vi "Create_Trajectory_Using_PathfinderDifferential_NAT.vi"() -> ()   [LabVIEW 2019]
uses:
  <vilib>/Rock Robotics/WPI/ThirdParty/JAS_Junk/JaciPathFinderLib/VIs/Waypoint.ctl
  <vilib>/Rock Robotics/WPI/ThirdParty/JAS_Junk/TrajLib/TRAJ_STATE.ctl
  <vilib>/Rock Robotics/WPI/ThirdParty/JAS_Junk/TrajLib/POSE2D.ctl
  <vilib>/Rock Robotics/WPI/ThirdParty/JAS_Junk/TrajLib/TRANSLATION2D.ctl
  <vilib>/Rock Robotics/WPI/ThirdParty/JAS_Junk/TrajLib/ROTATION2D.ctl
  <vilib>/Utility/miscctls.llb/LVCursorListTypeDef.ctl
  <vilib>/Rock Robotics/WPI/ThirdParty/JAS_Junk/TrajLib/UTIL_PATHFINDER_CONFIG.ctl
  <vilib>/Rock Robotics/WPI/ThirdParty/JAS_Junk/TrajLib/DISPLAY_WAYPOINT.ctl
  <vilib>/Utility/inputDevices.llb/mouseAcquire.vi
  <vilib>/Rock Robotics/WPI/ThirdParty/JAS_Junk/JaciPathFinderLib/Pathfinder.lvlib
  <vilib>/Rock Robotics/WPI/ThirdParty/JAS_Junk/TrajLib/Trajectory_Library.lvlib
panel:
  out "CursIdx":i32
  out "Cursor Update Mode":i32=1
  out "Angle":dbl
  out "Scrolling":i32
  out "Index":i32
  in  "End Program":bool
  in  "Tab Control":T1(tab)
  in  "max_velocity":dbl=58.0
  in  "max_acceleration":dbl=65.0
  in  "max_jerk":dbl=70.0
  in  "wheelbase_width":dbl=20.866
  in  "Real max\n speed":dbl=65.0
  out "Position":cluster{dbl[], dbl[]}[](graph)
  in  "Waypoints":T2[](array[typedef])=[{"x"=15.0, "y"=105.0, "angle"=-45.0}, {"x"=105.0, "y"=65.0, "angle"=0.0}, {"x"=210.0, "y"=106.0, "angle"=45.0}]
  in  "Path Results\ndT":dbl=0.02 format="%7.3f"
  in  "sample_count":i32=100000
  out "Path calculation error":errorcluster
  out "Complete,\nReady to \nSave file":bool
  out "Path \nSpeed > \nMax":bool
  out "max speed":dbl
  in  "Remove Cursor":bool
  in  "Add Cursor":bool
  in  "Calculate\nPath":bool
  out "Path Data":cluster{dbl[], dbl[]}[](graph)
  out "Traj States\nSize":i32
  out "Trajectory States":T3[](array[typedef]) {"POSE"."ROTATION"."SIN" format="%13.4f"; "POSE"."ROTATION"."COS" format="%13.4f"; "POSE"."ROTATION"."VALUE" format="%13.4f"; "POSE"."TRANSLATION"."Y" format="%14.3f"; "POSE"."TRANSLATION"."X" format="%14.3f"}
  out "File Saved\nWithout\nError":bool
  in  "Trajectory Type":enum32{"Radio Selection 1", "Radio Selection 2"}(radio)
  out "File Creation\nError":errorcluster
  in  "Trajectory File Comment":string
  in  "Trajectory File Name":path
  in  "CreateCmdList":bool
  # "Create trajectory using \"Jaci's Pathfinder\"  (Display for differential drive robot)"
  # "Instructions:\n----------------  \nThis utility will create a trajectory,, show the data on the various tabs, and optionally write a \"robot relative\" trajectory to a \nfile. To use this utility:\n\n1) Read all of these instructions!\n2) Define the Robot Data. on the \"Robot Data\" tab.\n3) Define the \"Path Definition\" on the \"Define / Create Trajectory\" tab.  These are the beginning and ending positions/headings, and \n     internal positions/headings.\n4) Define the time increment.  0.020 is chosen since that matches the normal robot loop time.\n5) Define \"sample count\".  This is an internal PathFinder variable.  Leaving the value as default should work correctly.  Making \n    the value a little smaller will speed the program up a little.\n6) Press the \"Calculate Path\".  If a good path was calculated it will be displayed on the \"Field Position tab, and the \"Complete, \n    Ready to Save\" indicator will light.  The path can be recalculated many times before performing any other action.\n\nAfter a Path has been calculated, the \"trajectory can be written to a file.  The absolute path is converted to a robot relative \ntrajectory.  To do this:\n1) Enter a comment to be included in the file.  Anything can be entered.\n2) Select the file name.\n3) Select the type of trajectory to save, absolute or relative.\n4) Press \"Create Trajectory File\"  If an error occurs it will be displayed in the File Creation Error indicator.\n\nNotes:\n---------\n- All the robot parameters, path, and field dimensions are in INCHES, and DEGREES.  The resulting trajectory is converted to \n   METERS, and RADIANS to match the rest of this library!\n- The pathfinder path generation logic doesn't account distribution of speed to the left and right wheels.  As a result the \n   maximum speed can be exceeded.If this happens, but Path Speed > Max light will light and Ready to Execute will not \n   light.  Lower the maximum speed in the Robot Data tab and recalulate the path.  (CURRENTLY THIS LOGIC IS NOT COMPLETE.)\n- 2019 playing field size - width: 26 ft 11.25 In = 323.25 in , length: 52 ft 5.25 in = 629.25 in  (I didn't verify this for the 2020 version.)"
  # "ROBOT DATA"
  # "INCHES/SEC"
  # "INCHES/SEC"
  # "INCHES/SEC^2"
  # "INCHES/SEC^3"
  # "Simulated robot wheelbase is: 20.866"
  # "INCHES"
  # "Simulated robot max speed is: 68.266"
  # "SEC"
  # "PATH DEFINITION"
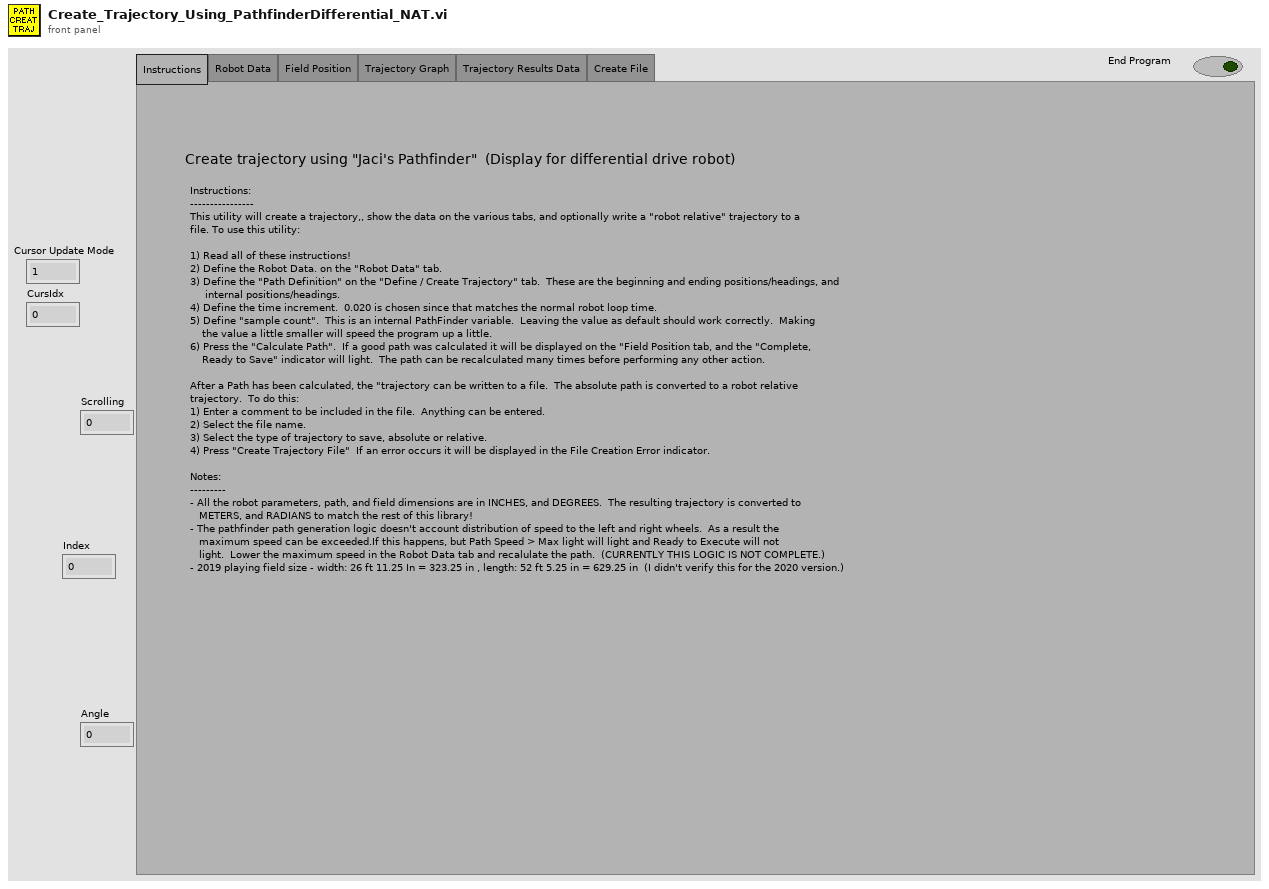
[diagram p1: front panel]
types:
  T1 = enum32{"Instructions", "Robot Data", "Field Position", "Trajectory Graph", "Trajectory Results Data", "Create File"}
  T2 = typedef "Pathfinder.lvlib/Waypoint.ctl" = cluster{"x":dbl, "y":dbl, "angle":dbl}
  T3 = typedef "Trajectory_Library.lvlib/TRAJ_STATE.ctl" = cluster{"TimeSeconds":dbl, "Velocity":dbl, "Acceleration":dbl, "POSE":T4, "Curvature":dbl}
  T4 = typedef "Trajectory_Library.lvlib/POSE2D.ctl" = cluster{"TRANSLATION":T5, "ROTATION":T6}
  T5 = typedef "Trajectory_Library.lvlib/TRANSLATION2D.ctl" = cluster{"X":dbl, "Y":dbl}
  T6 = typedef "Trajectory_Library.lvlib/ROTATION2D.ctl" = cluster{"VALUE":dbl, "COS":dbl, "SIN":dbl}
  T7 = typedef "LVCursorListTypeDef.ctl" = cluster{"Name":string, "Color":u32, "Style":u8, "Point Style":u8, "Name Visible":bool, "Allow Drag":bool, "Cursor Mode":u32, "Plot":i32, "Index":i32, "Position":cluster{"X":dbl, "Y":dbl}, "X Scale":u32, "Y Scale":u32, "Watch Plots":i32[], "Watch All Plots":bool, "Plot Area":i32, "Label Offset":cluster{"X":dbl, "Y":dbl}}[]
  T8 = typedef "Trajectory_Library.lvlib/DISPLAY_WAYPOINT.ctl" = cluster{"X":dbl, "Y":dbl, "ANGLE":dbl}
  T9 = cluster{"Name":string, "Color":u32, "Style":u8, "Point Style":u8, "Name Visible":bool, "Allow Drag":bool, "Cursor Mode":u32, "Plot":i32, "Index":i32, "Position":cluster{"X":dbl, "Y":dbl}, "X Scale":u32, "Y Scale":u32, "Watch Plots":i32[], "Watch All Plots":bool, "Plot Area":i32, "Label Offset":cluster{"X":dbl, "Y":dbl}}
  T10 = typedef "Trajectory_Library.lvlib/UTIL_PATHFINDER_CONFIG.ctl" = cluster{"PathfinderType - 0 tank 1 serve":i32, "PathMaxVelocity - inches per sec":dbl, "MaxAcceleration - inches per sec2":dbl, "MaxJerk--Inches per sec2":dbl, "TimeDelta-Seconds":dbl, "SampleCount":i32, "WheelbaseWidth-inches":dbl, "WheelbaseDepth-inches":dbl, "SwerveType":i32, "ActualMaxVelocity-inches per sec":dbl}
  T11 = cluster{"Horizontal":i32, "Vertical":i32, "Scrolling":i32}
  T12 = typedef "Trajectory_Library.lvlib/TRAJECTORY.ctl" = cluster{"TotalTImeSecs":dbl, "States":T3[]}
  T13 = typedef "Pathfinder.lvlib/Segment.ctl" = cluster{"dt":dbl, "x":dbl, "y":dbl, "position":dbl, "velocity":dbl, "acceleration":dbl, "jerk":dbl, "heading":dbl}
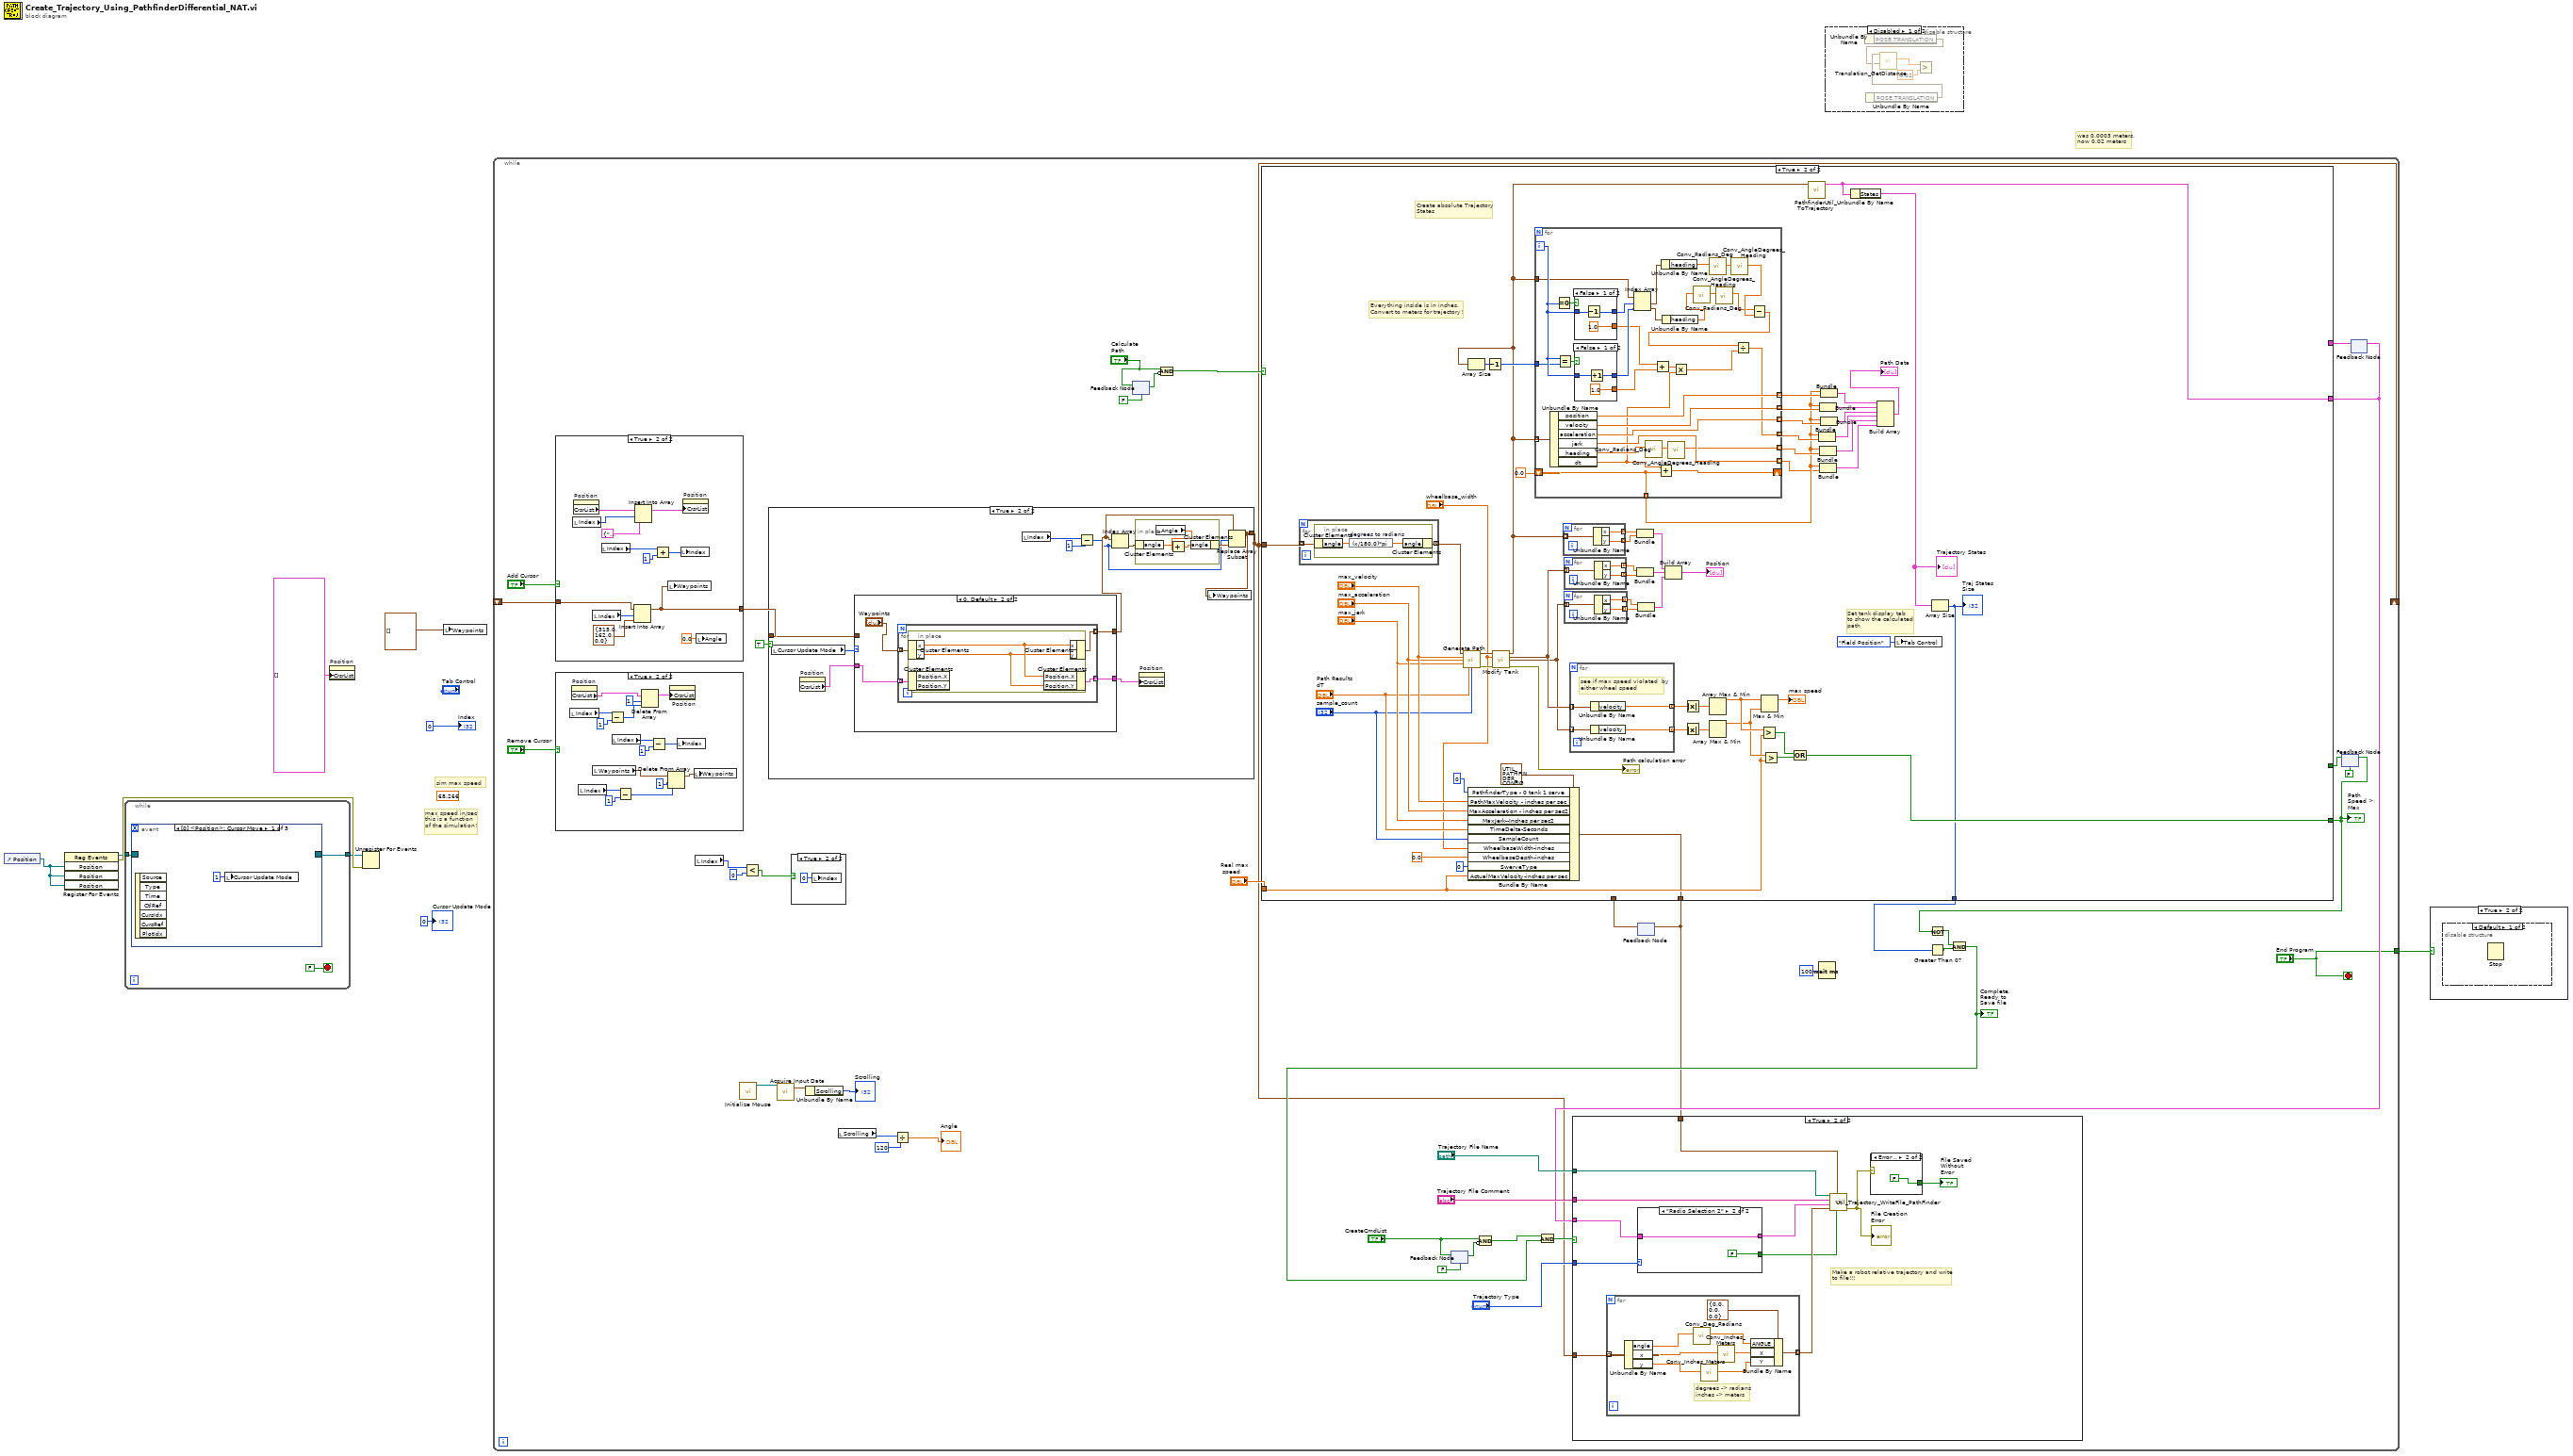
[diagram p0: block diagram]
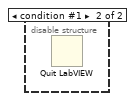
[diagram p3: hidden frame]
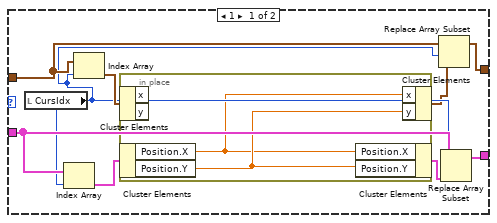
[diagram p5: hidden frame]
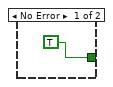
[diagram p9: hidden frame]
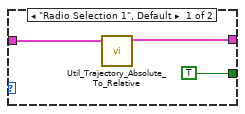
[diagram p10: hidden frame]
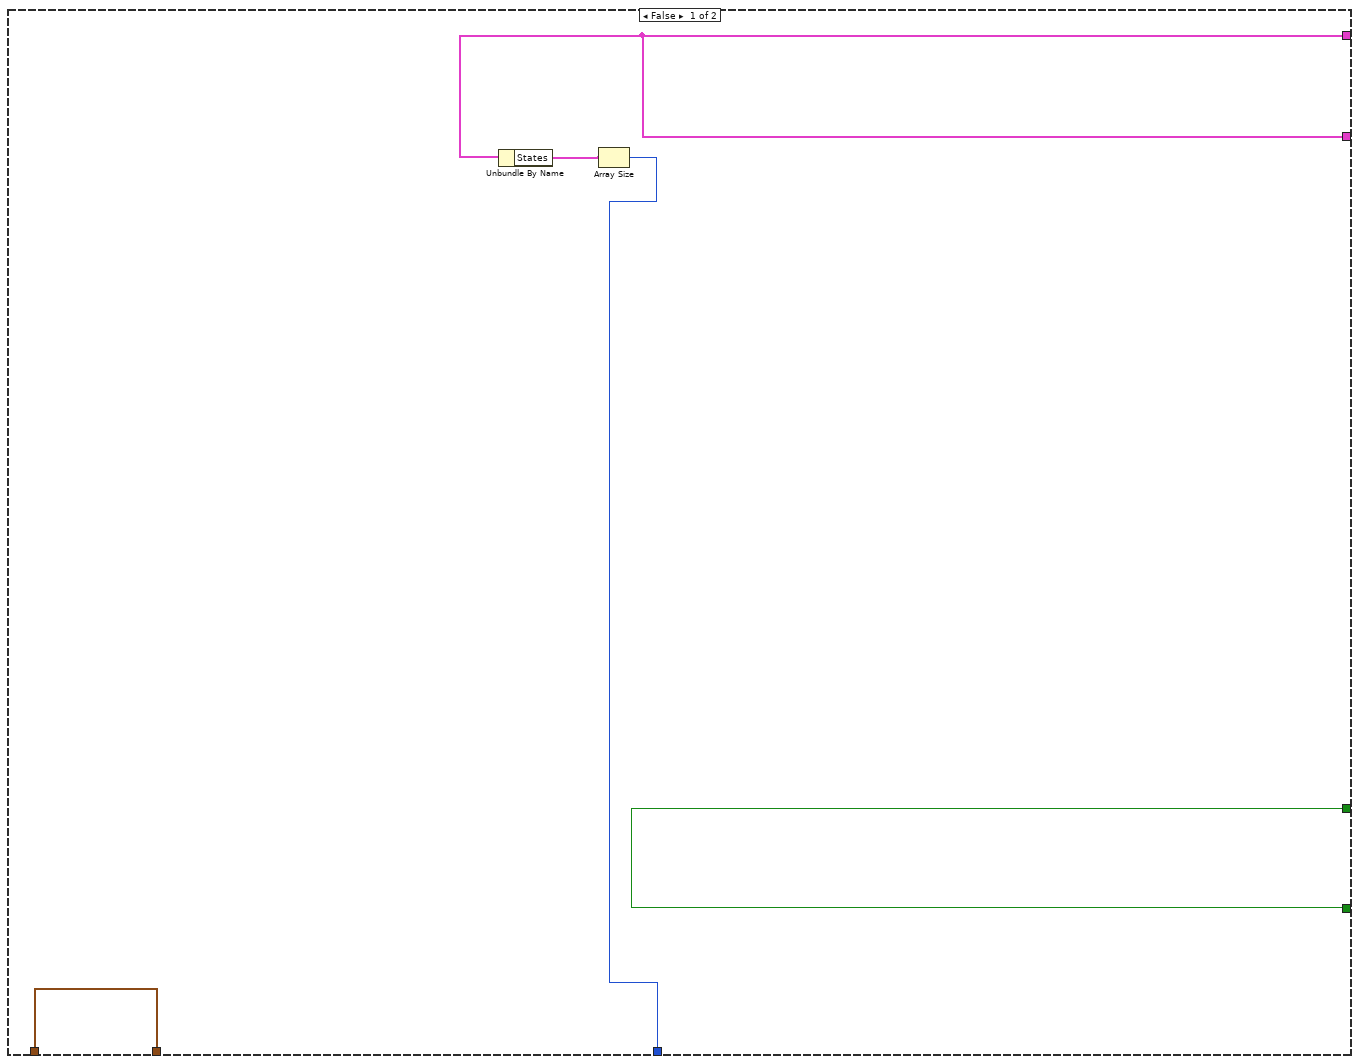
[diagram p12: hidden frame]
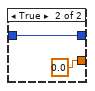
[diagram p13: hidden frame]
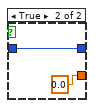
[diagram p14: hidden frame]
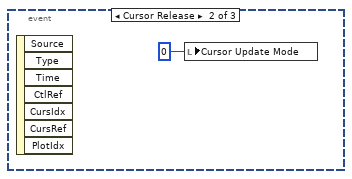
[diagram p15: hidden frame]
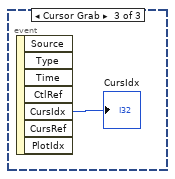
[diagram p16: hidden frame]
diagram:
  (unwired) 68.266 ("x")
  # "was 0.0003 meters.\nnow 0.02 meters"
  # "sim max speed"
  # "max speed in/sec\nthis is a function\nof the simulation!"
  n1 = control-ref of="Position"() -> (w4:refnum<vi>)
  n2 = register-events(w4, w4, w4) -> (reference out=w5:refnum<event-registration>, error out=w7:errorcluster)  [unwired: 2 in]
  n3 = while {
    tunnel: w5 -> [w12]
    tunnel: [w11] -> w6
    stop <- FALSE stop-if-true
    n4 = event shown="[0] <Position>: Cursor Move" {
      selector: w12 -> [_ _ _]
      dyn-events: [_ _ _] -> w11
      timeout: _ -> [_ _ _]
      event Cursor Move {
        n5 = event-data() -> ()  [unwired: 1 in, 7 out]
        n6 = local write "Cursor Update Mode"(1 ("Cursor Update Mode")) -> ()
      }
      event Cursor Release {
        n7 = event-data() -> ()  [unwired: 1 in, 7 out]
        n8 = local write "Cursor Update Mode"(0 ("Wapoint Update Mode")) -> ()
      }
      event Cursor Grab {
        n9 = event-data() -> ("CursIdx"=→"CursIdx":i32)  [unwired: 1 in, 6 out]
      }
    }
  }
  n10 = property on="Position" class="XYGraph (strict)"("CrsrList"=T7 [] ("Cursor List")) -> ()  [unwired: 2 in, 2 out]
  n11 = Unregister For Events(event registration refnum=w6, error in=w7) -> ()  [unwired: 1 out]
  n12 = local write "Waypoints"(T2[] [] ("Waypoints")) -> ()
  n13 = while {
    tunnel: ["End Program"] -> w9
    shift-right: [w17] -> _
    shift-left: _ -> [w22]
    stop <- "End Program" stop-if-true
    n14 = case shown="True" "Add Cursor" {
      tunnel: w22 -> [w136 w140]
      tunnel: [w136 w138] -> w18
      frame False {
      }
      frame True {
        n15 = local read "Index"() -> (w146:i32)
        n16 = property on="Position" class="XYGraph (strict)"() -> ("CrsrList"=w148:T7)  [unwired: 2 in, 2 out]
        n17 = local read "Index"() -> (w142:i32)
        n18 = local read "Index"() -> (w144:i32)
        n19 = Insert Into Array(array=w140, index=w142, new element=T2 {"x"=315.0, "y"=162.0, "angle"=0.0} ("new element/subarray")) -> (w138:T2[])
        n20 = Insert Into Array(array=w148, index=w146, new element=T9 {"Name"="Cursor", "Color"=5635906, "Style"=4, "Point Style"=2, "Name Visible"=FALSE, "Allow Drag"=TRUE, "Cursor Mode"=0, "Plot"=0, "Index"=0, "Position"={"X"=315.0, "Y"=162.0}, "X Scale"=0, "Y Scale"=0, "Watch Plots"=[], "Watch All Plots"=FALSE, "Plot Area"=0, "Label Offset"={"X"=0.0, "Y"=0.0}} ("new element/subarray")) -> (w147:T7)
        n21 = Add(x=w144, y=1) -> (x+y=w143:i32)
        n22 = local write "Waypoints"(w138) -> ()
        n23 = local write "Index"(w143) -> ()
        n24 = property on="Position" class="XYGraph (strict)"("CrsrList"=w147) -> ()  [unwired: 2 in, 2 out]
        n25 = local write "Angle"(0.0 ("Angle")) -> ()
      }
    }
    n26 = case shown="True" "Remove Cursor" {
      frame False {
      }
      frame True {
        n27 = local read "Index"() -> (w104:i32)
        n28 = property on="Position" class="XYGraph (strict)"() -> ("CrsrList"=w99:T7)  [unwired: 2 in, 2 out]
        n29 = local read "Index"() -> (w103:i32)
        n30 = local read "Waypoints"() -> (w95:T2[])
        n31 = Subtract(x=w104, y=1) -> (x-y=w101:i32)
        n32 = local read "Index"() -> (w107:i32)
        n33 = Subtract(x=w103, y=1) -> (x-y=w97:i32)
        n34 = Delete From Array(array=w99, length=1, index=w101) -> (array with subset deleted=w98:T7)  [unwired: 1 out]
        n35 = Subtract(x=w107, y=1) -> (x-y=w108:i32)
        n36 = Delete From Array(array=w95, length=1, index=w97) -> (array with subset deleted=w94:T2[])  [unwired: 1 out]
        n37 = property on="Position" class="XYGraph (strict)"("CrsrList"=w98) -> ()  [unwired: 2 in, 2 out]
        n38 = local write "Index"(w108) -> ()
        n39 = local write "Waypoints"(w94) -> ()
      }
    }
    n40 = local read "Index"() -> (w21:i32)
    n41 = call <vilib>:"Initialize Mouse.vi"() -> ("device ID"=w28:refnum<k1>)  [unwired: 10 in, 1 out]
    n42 = Less?(x=w21, y=0) -> (x < y?=w19:bool)
    n43 = case shown="True" TRUE {
      tunnel: w18 -> [w57 w67]
      tunnel: [w57 w58] -> w17
      frame False {
      }
      frame True {
        n44 = local read "Cursor Update Mode"() -> (w68:i32)
        n45 = property on="Position" class="XYGraph (strict)"() -> ("CrsrList"=w66:T7)  [unwired: 2 in, 2 out]
        n46 = case shown="0, Default" w68 {
          tunnel: w66 -> [w75 w86]
          tunnel: w67 -> [w78 _]
          tunnel: [w77 w85] -> w61
          tunnel: [w73 w84] -> w65
          frame 1 {
            n47 = local read "CursIdx"() -> (w74:i32)
            n48 = Index Array(array=w75, index=w74) -> (element=w80:T9)
            n49 = Index Array(array=w78, index=w74) -> (element=w79:T2)
            n50 = in-place {
              n51 = in-place-cluster #1(w79) -> ()  [unwired: 2 out]
              n52 = in-place-cluster #2(w80) -> ("Position.X"=w81:dbl, "Position.Y"=w82:dbl)
              n53 = in-place-cluster #2("Position.X"=w81, "Position.Y"=w82) -> (w76:T9)
              n54 = in-place-cluster #1("x"=w81, "y"=w82) -> (w72:T2)
            }
            n55 = Replace Array Subset(array=w78, new element=w72, index=w74) -> (w77:T2[])
            n56 = Replace Array Subset(array=w75, new element=w76, index=w74) -> (w73:T7)
          }
          frame 0, Default {
            n57 = for {
              tunnel: w86 -> [w90] mode=indexing
              tunnel: "Waypoints" -> [w89] mode=indexing
              tunnel: [w88] -> w85 mode=indexing
              tunnel: [w87] -> w84 mode=indexing
              n58 = in-place {
                n59 = in-place-cluster #3(w89) -> ("x"=w92:dbl, "y"=w91:dbl)
                n60 = in-place-cluster #4(w90) -> ()  [unwired: 2 out]
                n61 = in-place-cluster #4("Position.X"=w92, "Position.Y"=w91) -> (w87:T9)
                n62 = in-place-cluster #3("x"=w92, "y"=w91) -> (w88:T2)
              }
            }
          }
        }
        n63 = local read "Index"() -> (w60:i32)
        n64 = Subtract(x=w60, y=1) -> (x-y=w59:i32)
        n65 = Index Array(array=w61, index=w59) -> (element=w62:T2)
        n66 = in-place {
          n67 = in-place-cluster #5(w62) -> ("angle"=w71:dbl)
          n68 = local read "Angle"() -> (w70:dbl)
          n69 = Add(x=w70, y=w71) -> (x+y=w69:dbl)
          n70 = in-place-cluster #5("angle"=w69) -> (w64:T2)
        }
        n71 = property on="Position" class="XYGraph (strict)"("CrsrList"=w65) -> ()  [unwired: 2 in, 2 out]
        n72 = Replace Array Subset(array=w61, new element=w64, index=w59) -> (w58:T2[])
        n73 = local write "Waypoints"(w58) -> ()
      }
    }
    n74 = call-poly <vilib>:"Acquire Input Data.vi"("device ID"=w28) -> ("axis info"=w27:T11)  [unwired: 15 in, 3 out]
    n75 = case shown="True" w19 {
      frame False {
      }
      frame True {
        n76 = local write "Index"(0 ("Index")) -> ()
      }
    }
    n77 = Unbundle By Name(w27) -> ("Scrolling"=→"Scrolling":i32)
    n78 = local read "Scrolling"() -> (w23:i32)
    n79 = Divide(x=w23, y=120) -> (x/y=→"Angle":dbl)
    n80 = feedback #6(FALSE ("CreateCmdList")) -> (w39:bool)
    n81 = feedback-in #6("Calculate\nPath") -> ()
    n82 = Compound Arithmetic op=AND("Calculate\nPath", invert w39) -> (w36:bool)
    n83 = feedback-in #7("CreateCmdList") -> ()
    n84 = feedback #7(FALSE ("CreateCmdList")) -> (w42:bool)
    n85 = Compound Arithmetic op=AND("CreateCmdList", invert w42) -> (w41:bool)
    n86 = feedback #8() -> (w31:T10)  [unwired: 1 in]
    n87 = Wait (ms)(milliseconds to wait=u32 100) -> ()  [unwired: 1 out]
    n88 = feedback #9(FALSE) -> (w54:bool)
    n89 = feedback #10() -> (w50:T12)  [unwired: 1 in]
    n90 = case shown="True" w36 {
      tunnel: "Real max\n speed" -> [_ w158]
      tunnel: [w153 w199] -> w51
      tunnel: w54 -> [w153 _]
      tunnel: w17 -> [_ w198]
      tunnel: [w150 w175] -> w45
      tunnel: w50 -> [w150 _]
      tunnel: [w152 w190] -> w44
      tunnel: [w149 w154] -> w32
      tunnel: w31 -> [w149 _]
      frame False {
        n91 = Unbundle By Name(w150) -> ("States"=w151:T3[])
        n92 = Array Size(array=w151) -> (size(s)=w152:i32)
      }
      frame True {
        # "Everything inside is in inches.\nConvert to meters for trajectory!"
        # "Create absolute Trajectory\nStates"
        # "Set tank display tab\nto show the calculated\npath"
        n93 = for {
          tunnel: w198 -> [w220] mode=indexing
          tunnel: [w219] -> w212 mode=indexing
          n94 = in-place {
            n95 = in-place-cluster #11(w220) -> ("angle"=w222:dbl)
            n96 = expression code="(x/180.0)*pi" "degrees to radians"(w222) -> (w221:dbl)
            n97 = in-place-cluster #11("angle"=w221) -> (w219:T2)
          }
        }
        n98 = call <vilib>:"Generate Path.vi"("path"=w212, "max_velocity"="max_velocity", "max_acceleration"="max_acceleration", "max_jerk"="max_jerk", "dt (.001)"="Path Results\ndT", "sample_count (100000)"="sample_count") -> ("Segments"=w213:T13[], "error out"=w202:errorcluster)  [unwired: 8 in]
        n99 = Bundle By Name(cluster=T10 {"PathfinderType - 0 tank 1 serve"=0, "PathMaxVelocity - inches per sec"=0.0, "MaxAcceleration - inches per sec2"=0.0, "MaxJerk--Inches per sec2"=0.0, "TimeDelta-Seconds"=0.0, "SampleCount"=0, "WheelbaseWidth-inches"=0.0, "WheelbaseDepth-inches"=0.0, "SwerveType"=0, "ActualMaxVelocity-inches per sec"=0.0} ("UTIL_PATHFINDER_CONFIG"), "PathfinderType - 0 tank 1 serve"=0, "PathMaxVelocity - inches per sec"="max_velocity", "MaxAcceleration - inches per sec2"="max_acceleration", "MaxJerk--Inches per sec2"="max_jerk", "TimeDelta-Seconds"="Path Results\ndT", "SampleCount"="sample_count", "WheelbaseWidth-inches"="wheelbase_width", "WheelbaseDepth-inches"=0.0, "SwerveType"=0, "ActualMaxVelocity-inches per sec"=w158) -> (w154:T10)
        n100 = call <vilib>:"Modify Tank.vi"("Original"=w213, "wheelbase_width"="wheelbase_width", "error in"=w202) -> ("original"=w166:T13[], "left"=w197:T13[], "right"=w196:T13[], "error out"=→"Path calculation error":errorcluster)  [unwired: 9 in]
        n101 = Array Size(array=w166) -> (size(s)=w168:i32)
        n102 = Decrement(x=w168) -> (x-1=w167:i32)
        n103 = for {
          tunnel: w166 -> [w263] mode=indexing
          shift-right: [w261] -> _
          shift-left: 0.0 -> [w262]
          tunnel: [w262] -> w171 mode=indexing
          tunnel: [w254] -> w172 mode=indexing
          tunnel: [w260] -> w170 mode=indexing
          tunnel: [w259] -> w180 mode=indexing
          tunnel: [w258] -> w179 mode=indexing
          tunnel: [w257] -> w174 mode=indexing
          tunnel: [w240] -> w173 mode=indexing
          tunnel: w166 -> [w246]
          tunnel: w167 -> [w239]
          i -> [w251]
          n104 = Unbundle By Name(w263) -> ("position"=w257:dbl, "velocity"=w258:dbl, "acceleration"=w259:dbl, "jerk"=w260:dbl, "heading"=w256:dbl, "dt"=w242:dbl)
          n105 = Equal To 0?(x=w251) -> (x = 0?=w253:bool)
          n106 = Equal?(x=w251, y=w239) -> (x = y?=w252:bool)
          n107 = case shown="False" w253 {
            tunnel: w251 -> [w271 w272]
            tunnel: [1.0 0.0] -> w243
            tunnel: [w269 w272] -> w248
            frame False {
              n108 = Decrement(x=w271) -> (x-1=w269:i32)
            }
            frame True {
            }
          }
          n109 = case shown="False" w252 {
            tunnel: [1.0 0.0] -> w244
            tunnel: w251 -> [w265 w267]
            tunnel: [w264 w267] -> w247
            frame False {
              n110 = Increment(x=w265) -> (x+1=w264:i32)
            }
            frame True {
            }
          }
          n111 = Index Array(array=w246, index #1=w248, index #2=w247) -> (element #1=w250:T13, element #2=w249:T13)
          n112 = call <vilib>:"Conv_Radians_Deg.vi"("Radians"=w256) -> ("Degrees"=w255:dbl)  [unwired: 10 in]
          n113 = Add(x=w243, y=w244) -> (x+y=w245:dbl)
          n114 = Add(x=w242, y=w262) -> (x+y=w261:dbl)
          n115 = Unbundle By Name(w250) -> ("heading"=w236:dbl)
          n116 = Unbundle By Name(w249) -> ("heading"=w234:dbl)
          n117 = call <vilib>:"Conv_AngleDegrees_Heading.vi"("Degrees"=w255) -> ("Heading Degrees"=w254:dbl)  [unwired: 10 in]
          n118 = Multiply(x=w245, y=w242) -> (x*y=w241:dbl)
          n119 = call <vilib>:"Conv_Radians_Deg.vi"("Radians"=w234) -> ("Degrees"=w233:dbl)  [unwired: 10 in]
          n120 = call <vilib>:"Conv_Radians_Deg.vi"("Radians"=w236) -> ("Degrees"=w237:dbl)  [unwired: 10 in]
          n121 = call <vilib>:"Conv_AngleDegrees_Heading.vi"("Degrees"=w233) -> ("Heading Degrees"=w232:dbl)  [unwired: 10 in]
          n122 = call <vilib>:"Conv_AngleDegrees_Heading.vi"("Degrees"=w237) -> ("Heading Degrees"=w235:dbl)  [unwired: 10 in]
          n123 = Subtract(x=w232, y=w235) -> (x-y=w238:dbl)
          n124 = Divide(x=w238, y=w241) -> (x/y=w240:dbl)
        }
        n125 = for {
          tunnel: w166 -> [w225] mode=indexing
          tunnel: [w224] -> w209 mode=indexing
          tunnel: [w223] -> w210 mode=indexing
          n126 = Unbundle By Name(w225) -> ("x"=w224:dbl, "y"=w223:dbl)
        }
        n127 = for {
          tunnel: w197 -> [w231] mode=indexing
          tunnel: [w230] -> w203 mode=indexing
          tunnel: [w229] -> w204 mode=indexing
          n128 = Unbundle By Name(w231) -> ("x"=w230:dbl, "y"=w229:dbl)
        }
        n129 = for {
          tunnel: w196 -> [w228] mode=indexing
          tunnel: [w227] -> w205 mode=indexing
          tunnel: [w226] -> w206 mode=indexing
          n130 = Unbundle By Name(w228) -> ("x"=w227:dbl, "y"=w226:dbl)
        }
        n131 = for {
          tunnel: w197 -> [w218] mode=indexing
          tunnel: w196 -> [w217] mode=indexing
          tunnel: [w216] -> w195 mode=indexing
          tunnel: [w215] -> w193 mode=indexing
          # "see if max speed violated  by\neither wheel speed"
          n132 = Unbundle By Name(w218) -> ("velocity"=w216:dbl)
          n133 = Unbundle By Name(w217) -> ("velocity"=w215:dbl)
        }
        n134 = Bundle(w209, w210) -> (w211:cluster{dbl[], dbl[]})  [unwired: 1 in]
        n135 = Bundle(w203, w204) -> (w208:cluster{dbl[], dbl[]})  [unwired: 1 in]
        n136 = Bundle(w205, w206) -> (w207:cluster{dbl[], dbl[]})  [unwired: 1 in]
        n137 = Build Array(w211, w208, w207) -> (→"Position":cluster{dbl[], dbl[]}[])
        n138 = Absolute Value(x=w195) -> (abs(x)=w194:dbl[])
        n139 = Absolute Value(x=w193) -> (abs(x)=w192:dbl[])
        n140 = Array Max & Min(array=w194) -> (max value=w189:dbl)  [unwired: 3 out]
        n141 = Array Max & Min(array=w192) -> (max value=w188:dbl)  [unwired: 3 out]
        n142 = Max & Min(x=w189, y=w188) -> (max(x,y)=→"max speed":dbl)  [unwired: 1 out]
        n143 = Greater?(x=w189, y=w158) -> (0:w200:bool)
        n144 = Greater?(x=w188, y=w158) -> (0:w191:bool)
        n145 = Compound Arithmetic op=OR(w200, w191) -> (w199:bool)
        n146 = call <vilib>:"PathfinderUtil_ToTrajectory.vi"("Pathfinder Path"=w166) -> ("TRAJECTORY"=w175:T12)  [unwired: 10 in]
        n147 = Bundle(w171, w173) -> (w183:cluster{dbl[], dbl[]})  [unwired: 1 in]
        n148 = Bundle(w171, w172) -> (w182:cluster{dbl[], dbl[]})  [unwired: 1 in]
        n149 = Bundle(w171, w179) -> (w185:cluster{dbl[], dbl[]})  [unwired: 1 in]
        n150 = Bundle(w171, w170) -> (w169:cluster{dbl[], dbl[]})  [unwired: 1 in]
        n151 = Bundle(w171, w174) -> (w186:cluster{dbl[], dbl[]})  [unwired: 1 in]
        n152 = Bundle(w171, w180) -> (w184:cluster{dbl[], dbl[]})  [unwired: 1 in]
        n153 = Unbundle By Name(w175) -> ("States"=w177:T3[])
        "Trajectory States" <- w177
        n154 = Build Array(w186, w185, w184, w183, w182, w169) -> (→"Path Data":cluster{dbl[], dbl[]}[])
        n155 = local write "Tab Control"(T1."Field Position" ("Tab Control")) -> ()
        n156 = Array Size(array=w177) -> (size(s)=w190:i32)
        "Traj States\nSize" <- w190
      }
    }
    "Path \nSpeed > \nMax" <- w51
    n157 = feedback-in #8(w32) -> ()
    n158 = Not(x=w51) -> (.not. x?=w52:bool)
    n159 = Greater Than 0?(x=w44) -> (x > 0?=w53:bool)
    n160 = And(x=w52, y=w53) -> (x .and. y?=w46:bool)
    "Complete,\nReady to \nSave file" <- w46
    n161 = And(x=w41, y=w46) -> (x .and. y?=w47:bool)
    n162 = case shown="True" w47 {
      tunnel: "Trajectory File Name" -> [_ w119]
      tunnel: "Trajectory File Comment" -> [_ w118]
      tunnel: w45 -> [_ w114]
      tunnel: w17 -> [_ w117]
      tunnel: "Trajectory Type" -> [_ w113]
      tunnel: w32 -> [_ w109]
      frame False {
      }
      frame True {
        # "Make a robot relative trajectory and write\nto file!!!"
        n163 = for {
          tunnel: w117 -> [w135] mode=indexing
          tunnel: [w134] -> w116 mode=indexing
          # "degrees -> radians\ninches -> meters"
          n164 = Unbundle By Name(w135) -> ("angle"=w128:dbl, "x"=w133:dbl, "y"=w131:dbl)
          n165 = call <vilib>:"Conv_Deg_Radians.vi"("Degress"=w128) -> ("Radians"=w129:dbl)  [unwired: 10 in]
          n166 = call <vilib>:"Conv_Inches_Meters.vi"("INCH"=w131) -> ("Meters"=w130:dbl)  [unwired: 10 in]
          n167 = call <vilib>:"Conv_Inches_Meters.vi"("INCH"=w133) -> ("Meters"=w132:dbl)  [unwired: 10 in]
          n168 = Bundle By Name(cluster=T8 {"X"=0.0, "Y"=0.0, "ANGLE"=0.0} ("UTIL_WAYPOINT"), "ANGLE"=w129, "X"=w132, "Y"=w130) -> (w134:T8)
        }
        n169 = case shown="\"Radio Selection 2\"" w113 {
          tunnel: w114 -> [w124 w126]
          tunnel: [w123 w126] -> w115
          tunnel: [TRUE FALSE] -> w110
          frame "Radio Selection 1", Default {
            n170 = call <vilib>:"Util_Trajectory_Absolute_To_Relative.vi"("absTRAJECTORY"=w124) -> ("outputRelativeTRAJECTORY"=w123:T12)  [unwired: 10 in]
          }
          frame "Radio Selection 2" {
          }
        }
        n171 = call <vilib>:"Util_Trajectory_WriteFile_PathFinder.vi"("Trajectory Is Relative"=w110, "UTIL_PATHFINDER_CONFIG"=w109, "UtilityWayPoints"=w116, "TRAJECTORY"=w115, "Comment"=w118, "Trajectory File Name"=w119) -> ("error out"=w112:errorcluster)  [unwired: 5 in]
        "File Creation\nError" <- w112
        n172 = case shown="Error .." w112 {
          tunnel: [TRUE ("File Saved\nWithout\nError") FALSE ("File Saved\nWithout\nError")] -> w111
          frame No Error {
          }
          frame Error {
          }
        }
        "File Saved\nWithout\nError" <- w111
      }
    }
    n173 = feedback-in #9(w51) -> ()
    n174 = feedback-in #10(w45) -> ()
  }
  n175 = disable-structure shown="Disabled" {
    frame Disabled {
      n176 = Unbundle By Name() -> ("POSE.TRANSLATION"=w277:T5)  [unwired: 1 in]
      n177 = Unbundle By Name() -> ("POSE.TRANSLATION"=w278:T5)  [unwired: 1 in]
      n178 = call <vilib>:"Translation_GetDistance.vi"("other Translation"=w277, "In Translation"=w278) -> ("Distance"=w276:dbl)  [unwired: 9 in]
      n179 = Greater?(x=w276, y=0.02) -> (0:w274:bool)
    }
    frame Enabled {
    }
  }
  n180 = case shown="True" w9 {
    frame False {
    }
    frame True {
      n181 = disable-structure shown="Default" {
        frame condition #0 (active) {
          n182 = Stop() -> ()  [unwired: 1 in]
        }
        frame condition #1 {
          n183 = Quit LabVIEW() -> ()  [unwired: 1 in]
        }
      }
    }
  }
  "Index" <- 0 ("index")
  "Cursor Update Mode" <- 0
